vi "ListDirs.vi"(0 "root directory":path, 5 "include llbs? (no)":bool, 11 "error in (no error)":errorcluster) -> (4 "dup root":path, 8 "directory/llb list, including root":path[](array[path]), 15 "error out":errorcluster)   [LabVIEW 2011]
doc: "Recursively lists the directories, and optionally the llbs, contained in a root directory."
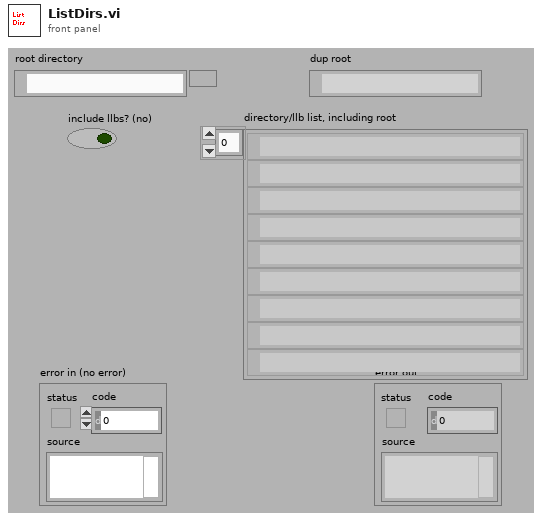
[diagram p1: front panel]
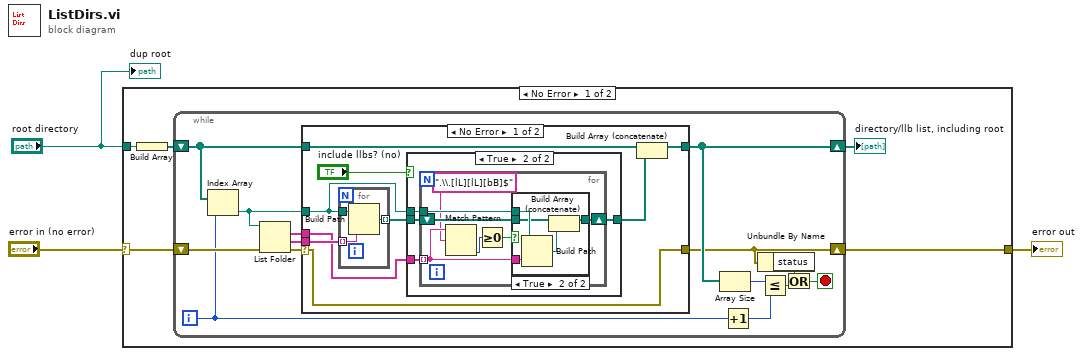
[diagram p0: block diagram]
diagram:
  n1 = case shown="No Error" "error in (no error)" {
    selector: "error in (no error)" -> [w8 w55]
    tunnel: [w6 w55] -> w2
    tunnel: "root directory" -> [w4 _]
    frame No Error {
      n2 = Build Array(w4) -> (w7:path[])
      n3 = while {
        shift-left: w8 -> [w22]
        shift-right: [w14] -> w6
        shift-left: w7 -> [w9]
        shift-right: [w15] -> w5
        i -> [w21]
        stop <- w16 stop-if-true
        n4 = Index Array(array=w9, index=w21) -> (element=w10:path)
        n5 = List Folder(path=w10, error in=w22) -> (filenames=w12:string[], folder names=w11:string[], error out=w13:errorcluster)  [unwired: 2 in, 1 out]
        n6 = case shown="No Error" w13 {
          selector: w13 -> [w29 w53]
          tunnel: w11 -> [w28 _]
          tunnel: w10 -> [w26 _]
          tunnel: w9 -> [w31 w54]
          tunnel: [w30 w54] -> w15
          tunnel: [w29 w53] -> w14
          tunnel: w12 -> [w24 _]
          frame No Error {
            n7 = for {
              tunnel: w28 -> [w51] mode=indexing
              tunnel: w26 -> [w52]
              tunnel: [w50] -> w27 mode=indexing
              n8 = Build Path(base path=w52, name or relative path=w51) -> (appended path=w50:path)
            }
            n9 = case shown="True" "include llbs? (no)" {
              tunnel: w27 -> [w32 w36]
              tunnel: w26 -> [_ w35]
              tunnel: [w32 w34] -> w25
              tunnel: w24 -> [_ w33]
              frame False {
              }
              frame True {
                n10 = for {
                  tunnel: w35 -> [w43]
                  tunnel: w33 -> [w40] mode=indexing
                  shift-right: [w41] -> w34
                  shift-left: w36 -> [w42]
                  n11 = Match Pattern(string=w40, regular expression=".\\.[lL][lL][bB]$") -> (offset past match=w38:i32)  [unwired: 1 in, 3 out]
                  n12 = Greater Or Equal To 0?(x=w38) -> (x >= 0?=w37:bool)
                  n13 = case shown="True" w37 {
                    tunnel: w43 -> [_ w49]
                    tunnel: w42 -> [w44 w46]
                    tunnel: [w44 w48] -> w41
                    tunnel: w40 -> [_ w45]
                    frame False {
                    }
                    frame True {
                      n14 = Build Path(base path=w49, name or relative path=w45) -> (appended path=w47:path)
                      n15 = Build Array (concatenate)(w46, w47) -> (w48:path[])
                    }
                  }
                }
              }
            }
            n16 = Build Array (concatenate)(w31, w25) -> (w30:path[])
          }
          frame Error {
          }
        }
        n17 = Array Size(array=w15) -> (size(s)=w20:i32)
        n18 = Increment(x=w21) -> (x+1=w19:i32)
        n19 = Unbundle By Name(w14) -> ("status"=w17:bool)
        n20 = Less Or Equal?(x=w20, y=w19) -> (x <= y?=w18:bool)
        n21 = Or(x=w17, y=w18) -> (x .or. y?=w16:bool)
      }
      "directory/llb list, including root" <- w5
    }
    frame Error {
    }
  }
  "error out" <- w2
  "dup root" <- "root directory"
